vi "CDS Library Unload.vi"(8 "error in (no error)":errorcluster, 11 "DMA Channel Testing in":refnum<class "DMA Channel Testing.lvclass">) -> (0 "error out":errorcluster, 3 "DMA Channel Testing out":refnum<class "DMA Channel Testing.lvclass">)   [LabVIEW 2019, in "DMA Channel Testing.lvclass"]
uses:
  DMA Channel Testing.lvclass
  DMA Channel Testing.lvclass/DMA Channel Testing.ctl
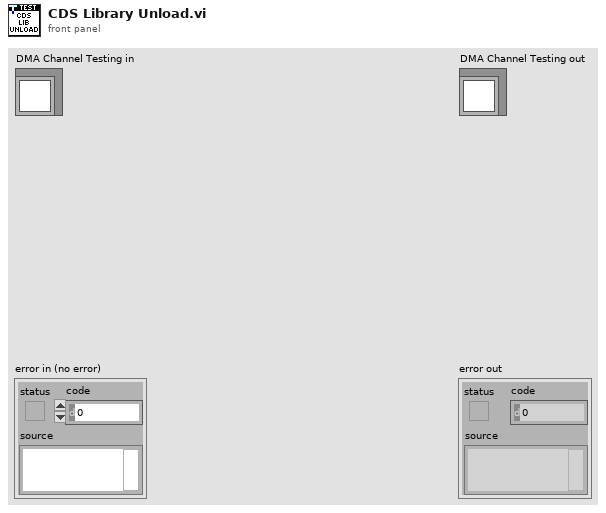
[diagram p1: front panel]
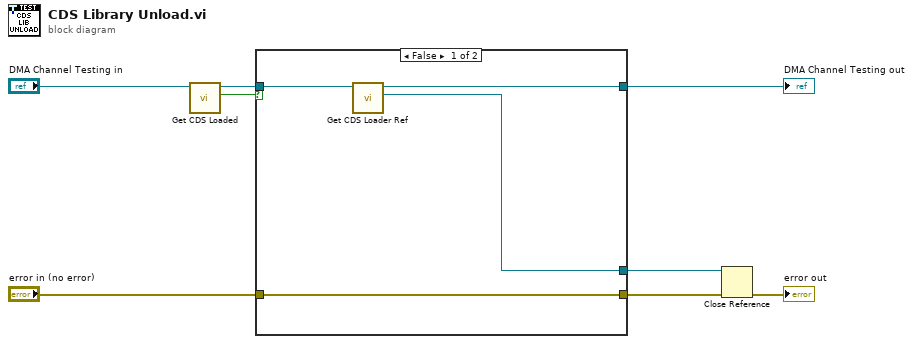
[diagram p0: block diagram]
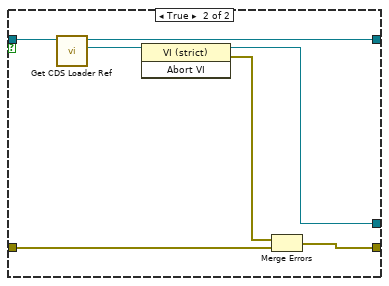
[diagram p2: hidden frame]
diagram:
  n1 = call "Get CDS Loaded.vi"("DMA Channel Testing in"="DMA Channel Testing in") -> ("CDS Loaded"=w7:bool, "DMA Channel Testing out"=w6:refnum<class "DMA Channel Testing.lvclass">)  [unwired: 9 in]
  n2 = case shown="False" w7 {
    tunnel: w6 -> [w12 w19]
    tunnel: [w11 w17] -> w1
    tunnel: "error in (no error)" -> [w9 w16]
    tunnel: [w10 w14] -> w2
    tunnel: [w9 w13] -> w4
    frame False {
      n3 = call "Get CDS Loader Ref.vi"("DMA Channel Testing in"=w12) -> ("CDS Loader Ref"=w10:refnum<vi>, "DMA Channel Testing out"=w11:refnum<class "DMA Channel Testing.lvclass">)  [unwired: 9 in]
    }
    frame True {
      n4 = call "Get CDS Loader Ref.vi"("DMA Channel Testing in"=w19) -> ("CDS Loader Ref"=w18:refnum<vi>, "DMA Channel Testing out"=w17:refnum<class "DMA Channel Testing.lvclass">)  [unwired: 9 in]
      n5 = invoke class="VI (strict)" method="Abort VI"(reference=w18) -> (reference out=w14:refnum<vi>, error out=w15:errorcluster)  [unwired: 2 in, 1 out]
      n6 = Merge Errors(w15, w16) -> (w13:errorcluster)
    }
  }
  "DMA Channel Testing out" <- w1
  n7 = Close Reference(reference=w2, error in (no error)=w4) -> (error out=→"error out":errorcluster)
